vi "Get Active VI Ref.vi"(8 "错误输入（无错误）":errorcluster) -> (0 "错误输出":errorcluster, 3 "Get Active VI Reference":refnum<vi>)   [LabVIEW 2012, in "Application.lvlib"]
uses:
  Application.lvlib
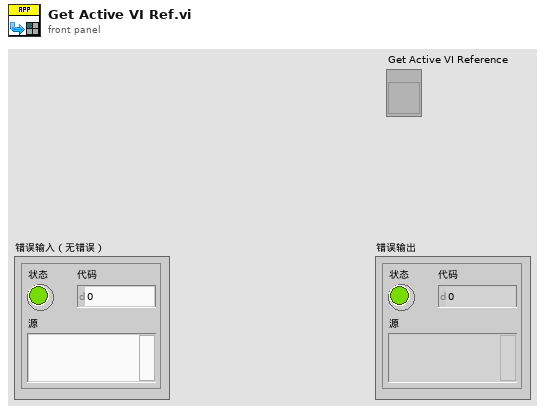
[diagram p1: front panel]
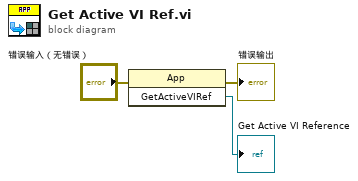
[diagram p0: block diagram]
diagram:
  n1 = invoke class="App" method="GetActiveVIRef"(error in="错误输入（无错误）") -> (error out=→"错误输出":errorcluster, "GetActiveVIRef"=→"Get Active VI Reference":refnum<vi>)  [unwired: 2 in, 1 out]
